vi "FP RT main.vi"() -> ()   [LabVIEW 2014]
uses:
  <vilib>/userdefined/High Color/IMAQdx.ctl
  <vilib>/myRIO/Instrument Drivers/Onboard IO/PWM/typedefs/PWM Reference.ctl
  <vilib>/myRIO/Common/Instrument Driver Framework/Utilities/typedefs/myRIO Generic Hardware Reference.ctl
  <vilib>/myRIO/Common/Instrument Driver Framework/Utilities/typedefs/Hardware Version Enum.ctl
  <vilib>/myRIO/Common/Instrument Driver Framework/Utilities/typedefs/myRIO v1.0 Reference.ctl
  <vilib>/myRIO/Common/Instrument Driver Framework/Utilities/typedefs/Generic FPGA Reference.ctl
  <vilib>/myRIO/Common/Instrument Driver Framework/myRIO v1.0/PWM/typedefs/PWM Channels Enum.ctl
  <vilib>/myRIO/Instrument Drivers/Onboard IO/PWM/typedefs/PWM Configuration.ctl
  <vilib>/userdefined/High Color/nirio_resource_hc.ctl
  <vilib>/myRIO/Instrument Drivers/Onboard IO/DIO/typedefs/DIO Reference.ctl
  <vilib>/myRIO/Common/Instrument Driver Framework/myRIO v1.0/DIO/typedefs/DIO Channels List.ctl
  <vilib>/myRIO/Common/Instrument Driver Framework/myRIO v1.0/DIO/typedefs/DIO Channels Enum.ctl
  <vilib>/myRIO/Instrument Drivers/Onboard IO/AI/typedefs/AI Reference.ctl
  <vilib>/myRIO/Common/Instrument Driver Framework/myRIO v1.0/AI/typedefs/AI Channels List.ctl
  <vilib>/myRIO/Common/Instrument Driver Framework/myRIO v1.0/AI/typedefs/AI Channels Enum.ctl
  <vilib>/myRIO/Common/Instrument Driver Framework/Utilities/typedefs/Analog Scaling Constants List.ctl
  <vilib>/myRIO/Common/Instrument Driver Framework/Utilities/typedefs/Analog Scaling Constants.ctl
  <vilib>/myRIO/Common/Instrument Driver Framework/myRIO v1.0/PWM/vis/myRIO v1.1 Open PWM.vi
  <vilib>/myRIO/Common/Instrument Driver Framework/myRIO v1.0/DIO/vis/myRIO v1.1 Open DIO.vi
  <vilib>/myRIO/Common/Instrument Driver Framework/myRIO v1.0/AI/vis/myRIO v1.1 Open AI.vi
  <vilib>/myRIO/Common/Instrument Driver Framework/Utilities/vis/Validate Channels.vi
  <vilib>/myRIO/Common/Instrument Driver Framework/myRIO v1.0/PWM/vis/myRIO v1.0 Reserve PWM.vi
  <vilib>/myRIO/Common/Instrument Driver Framework/myRIO v1.0/DIO/vis/myRIO v1.0 Reserve DIO.vi
  <vilib>/myRIO/Common/Instrument Driver Framework/myRIO v1.0/AI/vis/myRIO v1.0 Reserve AI.vi
  <vilib>/myRIO/Common/Instrument Driver Framework/myRIO v1.0/PWM/vis/myRIO v1.0 Close PWM.vi
  <vilib>/myRIO/Common/Instrument Driver Framework/myRIO v1.0/DIO/vis/myRIO v1.0 Close DIO.vi
  <vilib>/myRIO/Common/Instrument Driver Framework/myRIO v1.0/AI/vis/myRIO v1.0 Close AI.vi
  <vilib>/myRIO/Common/Instrument Driver Framework/myRIO v1.0/PWM/vis/myRIO v1.0 Build MUX Configuration PWM.vi
  <vilib>/myRIO/Common/Instrument Driver Framework/myRIO v1.0/Resource Manager/vis/myRIO v1.0 Reserve Channel List.vi
  <vilib>/myRIO/Common/Instrument Driver Framework/myRIO v1.0/DIO/vis/myRIO v1.0 Build MUX Configuration DIO.vi
  <vilib>/myRIO/Common/Instrument Driver Framework/myRIO v1.0/AI/vis/myRIO v1.0 Build MUX Configuration AI.vi
  <vilib>/myRIO/Common/Instrument Driver Framework/myRIO v1.0/PWM/vis/myRIO v1.0 Unreserve PWM.vi
  <vilib>/myRIO/Common/Instrument Driver Framework/myRIO v1.0/DIO/vis/myRIO v1.0 Unreserve DIO.vi
  <vilib>/myRIO/Common/Instrument Driver Framework/myRIO v1.0/AI/vis/myRIO v1.0 Unreserve AI.vi
  <vilib>/myRIO/Common/Instrument Driver Framework/myRIO v1.0/Resource Manager/vis/myRIO v1.0 Create Configuration List.vi
  <vilib>/myRIO/Common/Instrument Driver Framework/myRIO v1.0/Resource Manager/vis/myRIO v1.0 Reserve Channel.vi
  <vilib>/myRIO/Common/Instrument Driver Framework/myRIO v1.0/Resource Manager/vis/myRIO v1.0 Unreserve Channel.vi
  <vilib>/myRIO/Common/Instrument Driver Framework/myRIO v1.0/Resource Manager/vis/myRIO v1.0 Unreserve Channel List.vi
  <vilib>/myRIO/Common/Instrument Driver Framework/myRIO v1.0/Resource Manager/vis/myRIO v1.0 Build Mutex Name.vi
  <vilib>/Utility/VariantDataType/GetNumericInfo.vi
  <vilib>/Utility/error.llb/Error Cluster From Error Code.vi
  <vilib>/myRIO/Common/Instrument Driver Framework/myRIO v1.0/myRIO v1.1 Open.vi
  <vilib>/myRIO/Common/Instrument Driver Framework/myRIO v1.0/AI/vis/myRIO v1.0 Get Scaling Constants AI.vi
  <vilib>/myRIO/Common/Instrument Driver Framework/Utilities/vis/IO Manager.vi
  <vilib>/myRIO/Common/Instrument Driver Framework/Utilities/vis/Configuration Manager.vi
  <vilib>/myRIO/Common/Instrument Driver Framework/myRIO v1.0/myRIO v1.0 Close.vi
  <vilib>/myRIO/Common/Instrument Driver Framework/myRIO v1.0/Resource Manager/vis/myRIO v1.0 Configure IO.vi
  <vilib>/myRIO/Common/Instrument Driver Framework/myRIO v1.0/AI/vis/myRIO v1.0 Read AI.vi
  <vilib>/myRIO/Common/Instrument Driver Framework/myRIO v1.0/DIO/vis/myRIO v1.0 Write DIO.vi
  <vilib>/myRIO/Common/Instrument Driver Framework/myRIO v1.0/PWM/vis/myRIO v1.0 Write PWM.vi
  <vilib>/myRIO/Common/Instrument Driver Framework/myRIO v1.0/PWM/vis/myRIO v1.0 Shutdown PWM.vi
  <vilib>/myRIO/Common/Instrument Driver Framework/myRIO v1.0/DIO/vis/myRIO v1.0 Shutdown DIO.vi
  <vilib>/myRIO/Instrument Drivers/Onboard IO/AI/vis/myRIO AI Open.xnode
  <vilib>/myRIO/Instrument Drivers/Onboard IO/DIO/vis/myRIO DIO Open.xnode
  <vilib>/myRIO/Instrument Drivers/Onboard IO/PWM/vis/myRIO PWM Open.xnode
  <vilib>/vision/driver/NI_Vision_Acquisition_Software.lvlib
  <vilib>/myRIO/Instrument Drivers/Onboard IO/AI/AI.lvlib
  <vilib>/myRIO/Instrument Drivers/Onboard IO/DIO/DIO.lvlib
  <vilib>/myRIO/Instrument Drivers/Onboard IO/PWM/PWM.lvlib
panel:
  in  "Tab Control":T1(tab)
  out "BW Image":T2(plugin-control)
  in  "stop":bool
  out "Midbrain?":bool
  out "Rudder":dbl(knob) min=-45.0 max=45.0 step=1.0 scale=-45.0..45.0
  out "Speed":dbl(knob) min=-9.0 max=9.0 step=1.0 scale=-50.0..50.0
  out "Hindbrain?":bool
  out "Forebrain?":bool
  out "Battery Dead?":bool
  out "Complete?":bool=TRUE
  out "Arbiter Graph":cluster{dbl, dbl, dbl[]}(graph)
  in  "Session In":T3="cam0"
  out "Color Image":T2(plugin-control)
  out "Nb Circles":i32
  out "UDP Time Out?":bool
  in  "Tug letter":string="G"
  in  "Run?":bool
  in  "MSpeed":dbl(slide) scale=-50.0..50.0 scale format="%#.1g"
  in  "MHeading":dbl(slide) scale=-45.0..45.0 scale format="%_1f"
  in  "Manual?":bool
  out "Camera Data":T4(array[cluster])
  out "Boat Status":T5={"GPS"={"X pos"=0, "Y pos"=0, "Heading"=0.0}, "IR Sensors"=[{"Name"="Bow", "Angle"=0.0, "Distance"=0.0}], "MOT BAT"=7.2, "RIO BAT"=7.2}
  out "GPS?":bool
  out "Act Com":T6
  out "Forebrain ACT":dbl[](array[numeric])
  out "IR Sensors":T7(array[cluster])
  out "GPS":cluster{"X pos":i32, "Y pos":i32, "Heading":dbl}
  out "RED LED":bool
  out "GREEN LED":bool
  out "BLUE LED":bool
  in  "MDF":T8(array[cluster])=[{"Type"=enum."Start", "X"=250, "Y"=250, "Speed"=0, "Behaviors"=enum."Open Water Transit"}, {"Type"=enum."Waypoint", "X"=400, "Y"=100, "Speed"=20, "Behaviors"=enum."P-Wall Follow"}, {"Type"=enum."Waypoint", "X"=250, "Y"=250, "Speed"=20, "Behaviors"=enum."Open Water Transit"}, {"Type"=enum."Waypoint", "X"=250, "Y"=400, "Speed"=20, "Behaviors"=enum."Open Water Transit"}, {"Type"=enum."Waypoint", "X"=100, "Y"=400, "Speed"=20, "Behaviors"=enum."Open Water Transit"}, {"Type"=enum."End", "X"=250, "Y"=250, "Speed"=0, "Behaviors"=enum."Open Water Transit"}]
  out "Invalid Pos?":bool
  out "error out":errorcluster
  out "Forebrain Comd":T9
  out "size(s)":i32
  out "MDF Active":T8(array[cluster])
  # "To start the Tug, press the \">\" key in the tool bar.\n\nPress the Run? control to start the Mission.\n\nWhen complete the Complete? indicator will light.\n\nIf the Run? is not pressed again, the mission will start again.\n\nAlways press the STOP button to end the operation!!!!!!!!!!!!!"
  # "Press the Manual? button to control\nthe Tug from the sliders"
  # "Stuck indicates that\nthe boat is not moving."
  # "Enter the Letter\nof  your Tug"
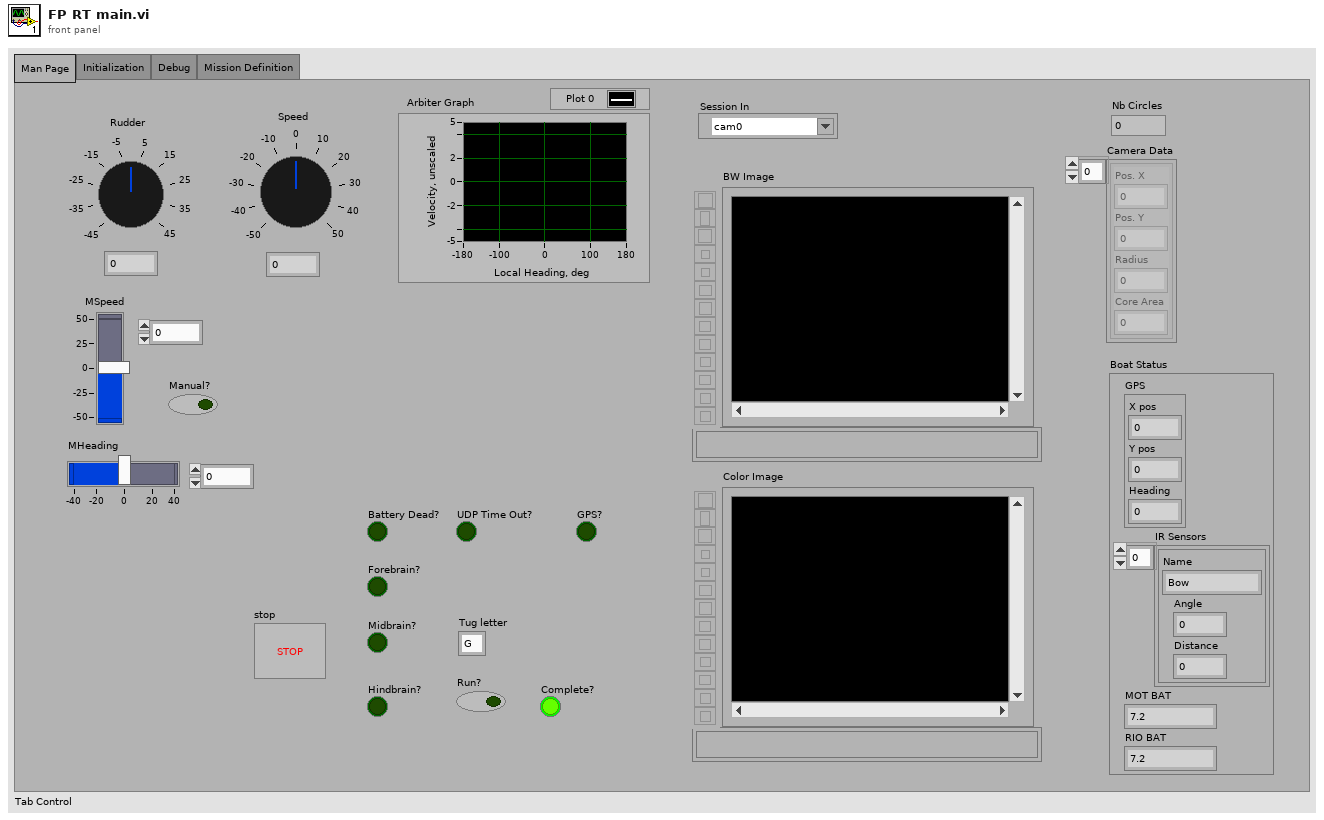
[diagram p1: front panel]
types:
  T1 = enum32{"Man Page", "Initialization", "Debug", "Mission Definition"}
  T2 = typedef "IMAQ Image.ctl" = refnum<image>
  T3 = typedef "IMAQdx.ctl" = refnum<k21>
  T4 = cluster{"Pos. X":i32, "Pos. Y":i32, "Radius":i32, "Core Area":i32}[]
  T5 = cluster{"GPS":cluster{"X pos":i32, "Y pos":i32, "Heading":dbl}, "IR Sensors":cluster{"Name":string, "Angle":dbl, "Distance":dbl}[], "MOT BAT":dbl, "RIO BAT":dbl}
  T6 = cluster{"Desired Local\nHeading":dbl, "Desired\nSpeed":dbl}
  T7 = cluster{"Name":string, "Angle":dbl, "Distance":dbl}[]
  T8 = cluster{"Type":enum16{"Start", "Waypoint", "End"}, "X":i32, "Y":i32, "Speed":i32, "Behaviors":enum16{"Open Water Transit", "P-Wall Follow", "S-Wall Follow", "Dock"}}[]
  T9 = cluster{"Behaviors":enum16{"Open Water Transit", "P-Wall Follow", "S-Wall Follow", "Dock"}, "Behavior\nVelocity":dbl}
  T10 = typedef "nirio_resource_hc.ctl" = tag
  T11 = typedef "Hardware Version Enum.ctl" = enum16{"Unknown", "myRIO-1900", "myRIO-1950"}
  T12 = typedef "Image Type" = u32
  T13 = enum16{"Open Water Transit", "P-Wall Follow", "S-Wall Follow", "Dock"}
  T14 = typedef "PWM.lvlib/PWM Reference.ctl" = cluster{"myRIO Reference":T15, "PWM Channels Enum":T18, "PWM Configuration":T19}
  T15 = typedef "myRIO Generic Hardware Reference.ctl" = cluster{"myRIO Model":T11, "myRIO Hardware Reference":T16}
  T16 = typedef "myRIO v1.0 Reference.ctl" = cluster{"Generic FPGA Reference":T17, "Allow multiple opens":bool}
  T17 = typedef "Generic FPGA Reference.ctl" = refnum<k20>
  T18 = typedef "PWM Channels Enum.ctl" = enum16{"Not Connected", "C/PWM0", "C/PWM1", "A/PWM0", "A/PWM1", "A/PWM2", "B/PWM0", "B/PWM1", "B/PWM2"}
  T19 = typedef "PWM.lvlib/PWM Configuration.ctl" = cluster{"Frequency":dbl, "Duty Cycle":dbl}
  T20 = typedef "DIO.lvlib/DIO Reference.ctl" = cluster{"myRIO Reference":T15, "DIO Channels List":T21}
  T21 = typedef "DIO Channels List.ctl" = T22[]
  T22 = typedef "DIO Channels Enum.ctl" = enum16{"Not Connected", "C/DIO0", "C/DIO1", "C/DIO2", "C/DIO3", "C/DIO4", "C/DIO5", "C/DIO6", "C/DIO7", "A/DIO0", "A/DIO1", "A/DIO2", "A/DIO3", "A/DIO4", "A/DIO5", "A/DIO6", "A/DIO7", "A/DIO8", "A/DIO9", "A/DIO10", "A/DIO11", "A/DIO12", "A/DIO13", "A/DIO14", "A/DIO15", "B/DIO0", "B/DIO1", "B/DIO2", "B/DIO3", "B/DIO4", "B/DIO5", "B/DIO6", "B/DIO7", "B/DIO8", "B/DIO9", "B/DIO10", "B/DIO11", "B/DIO12", "B/DIO13", "B/DIO14", "B/DIO15", "LED0", "LED1", "LED2", "LED3", "Button0"}
  T23 = typedef "AI.lvlib/AI Reference.ctl" = cluster{"myRIO Reference":T15, "AI Channels List":T24, "AI Scaling Constants List":T26}
  T24 = typedef "AI Channels List.ctl" = T25[]
  T25 = typedef "AI Channels Enum.ctl" = enum16{"Not Connected", "AudioIn/Left", "AudioIn/Right", "C/AI0", "C/AI1", "A/AI0", "A/AI1", "A/AI2", "A/AI3", "B/AI0", "B/AI1", "B/AI2", "B/AI3"}
  T26 = typedef "Analog Scaling Constants List.ctl" = T27[]
  T27 = typedef "Analog Scaling Constants.ctl" = cluster{"LSB Weight (Volts)":dbl, "Offset (Volts)":dbl, "Signed?":bool}
  T28 = cluster{"Obs Avoid Array":dbl[], "P-Wall Array":dbl[], "S-Wall Array":dbl[], "Unstuck Array":dbl[]}
  T29 = cluster{"regular expression":string, i32, i32, i32}
  T30 = cluster{"Behaviors":enum16{"Open Water Transit", "P-Wall Follow", "S-Wall Follow", "Dock"}, dbl}
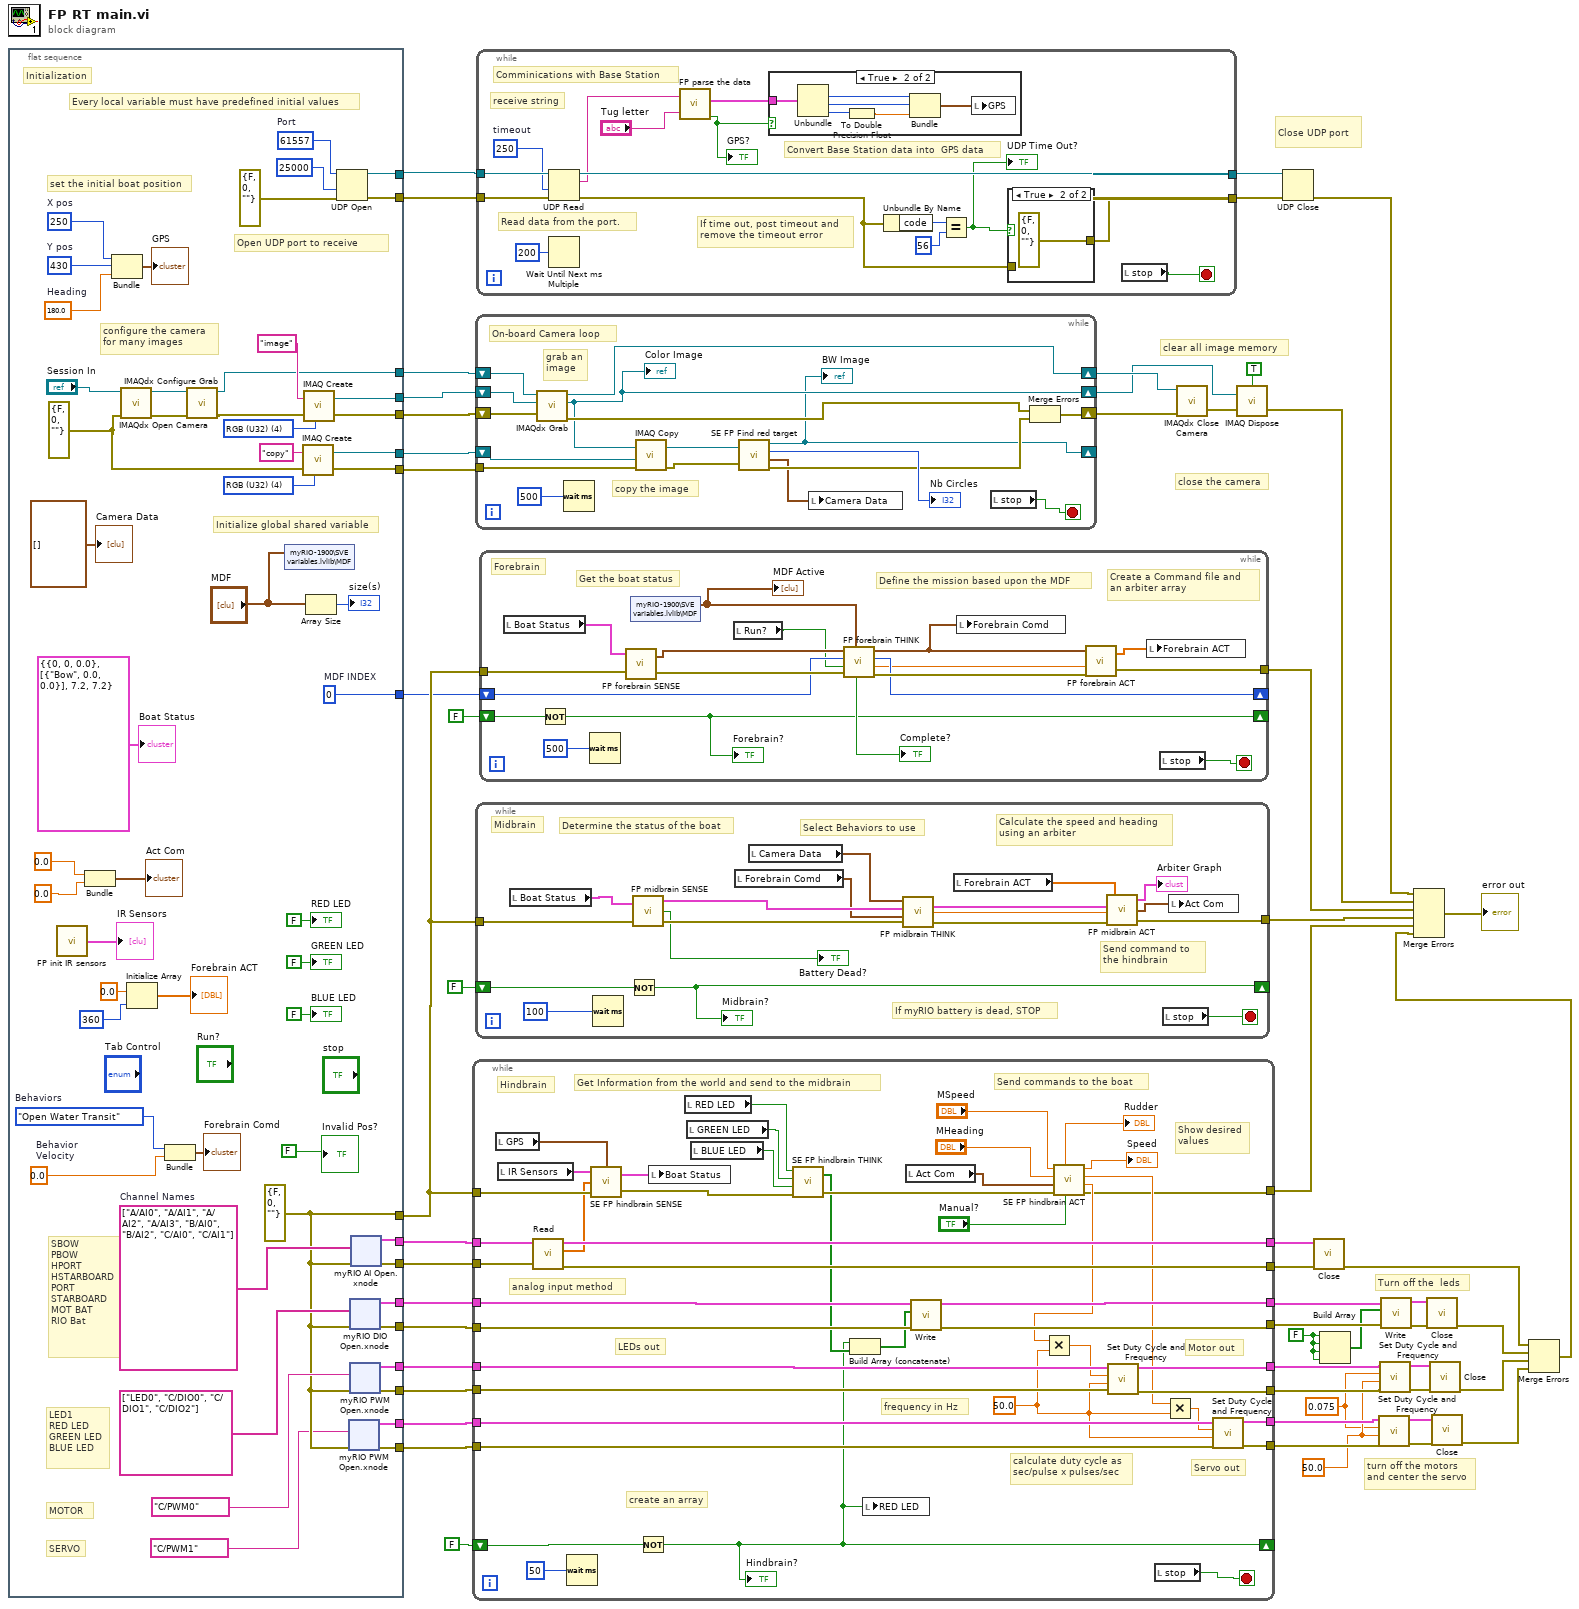
[diagram p0: block diagram]
diagram:
  w2 = 0.075
  w1 = FALSE
  w3 = 50.0
  # "Turn off the  leds"
  # "turn off the motors\nand center the servo"
  # "Close UDP port"
  # "clear all image memory"
  # "close the camera"
  n1 = flat-sequence {
    tunnel: [w68] -> w51
    tunnel: [w103] -> w48
    tunnel: [w94] -> w47
    tunnel: [w93] -> w46
    tunnel: [w92] -> w45
    tunnel: [w88] -> w38
    tunnel: [w87] -> w39
    tunnel: [w83] -> w33
    tunnel: [w82] -> w34
    tunnel: [w76] -> w31
    tunnel: [w75] -> w30
    tunnel: [w73] -> w26
    tunnel: [w72] -> w27
    tunnel: [w70] -> w25
    tunnel: [w69] -> w24
    tunnel: [w66] -> w23
    tunnel: [w65] -> w22
    frame #0 {
      w77 = tag[] ["A/AI0", "A/AI1", "A/AI2", "A/AI3", "B/AI0", "B/AI2", "C/AI0", "C/AI1"]  # Channel Names
      w79 = 430  # Y pos
      w80 = 250  # X pos
      w81 = 180.0  # Heading
      w86 = u16 61557  # Port
      w91 = T12 4 items=["Grayscale (U8)", "Grayscale (I16)", "Grayscale (SGL)", "Complex (CSG)", "RGB (U32)", "HSL (U32)", "RGB (U64)", "Grayscale (U16)"] ("Image Type")
      w89 = errorcluster {"status"=FALSE, "code"=0, "source"=""} ("error in")
      w99 = T12 4 items=["Grayscale (U8)", "Grayscale (I16)", "Grayscale (SGL)", "Complex (CSG)", "RGB (U32)", "HSL (U32)", "RGB (U64)", "Grayscale (U16)"] ("Image Type")
      w68 = errorcluster {"status"=FALSE, "code"=0, "source"=""} ("error out")
      w103 = 0  # MDF INDEX
      w107 = 0.0  # Behavior Velocity
      w102 = T13."Open Water Transit"  # Behaviors
      # "Initialize global shared variable"
      # "LED1\nRED LED\nGREEN LED\nBLUE LED"
      # "SERVO"
      # "MOTOR"
      # "SBOW\nPBOW\nHPORT\nHSTARBOARD\nPORT\nSTARBOARD\nMOT BAT\nRIO Bat"
      # "set the initial boat position"
      # "Open UDP port to receive"
      # "configure the camera\nfor many images"
      # "Every local variable must have predefined initial values"
      # "Initialization"
      n2 = call "FP init IR sensors.vi"() -> ("IR Sensors"=→"IR Sensors":T7)  [unwired: 1 in]
      n3 = Bundle(0.0, 0.0) -> (→"Act Com":cluster{dbl, dbl})  [unwired: 1 in]
      n4 = Bundle("X pos"=w80, "Y pos"=w79, "Heading"=w81) -> (→"GPS":cluster{"X pos":i32, "Y pos":i32, "Heading":dbl})  [unwired: 1 in]
      n5 = call <vilib>:"IMAQdx Open Camera.vi"("error in"=w89, "Session In"="Session In") -> ("error out"=w96:errorcluster, "Session Out"=w95:T3)  [unwired: 1 in, 7 out]
      n6 = Initialize Array(0.0 ("element"), 360 ("dimension size")) -> (→"Forebrain ACT":dbl[])
      n7 = Bundle("Behaviors"=w102, "Behavior\nVelocity"=w107) -> (→"Forebrain Comd":T9)  [unwired: 1 in]
      n8 = call <vilib>:"IMAQdx Configure Grab.vi"("error in"=w96, "Session In"=w95) -> ("error out"=w100:errorcluster, "Session Out"=w92:T3)  [unwired: 8 out]
      n9 = shared-variable "myRIO-1900\\SVE variables.lvlib\\MDF"("MDF") -> ()  [unwired: 1 in, 1 out]
      n10 = call "IMAQ Create"("Image Name"="copy", "Image Type"=w91, "error in (no error)"=w89) -> ("New Image"=w87:T2, "error out"=w88:errorcluster)  [unwired: 2 in]
      n11 = call "IMAQ Create"("Image Name"="image", "Image Type"=w99, "error in (no error)"=w100) -> ("New Image"=w93:T2, "error out"=w94:errorcluster)  [unwired: 1 in, 1 out]
      n12 = Array Size(array="MDF") -> (size(s)=→"size(s)":i32)
      n13 = UDP Open(8:errorcluster {"status"=FALSE, "code"=0, "source"=""} ("error in"), 9:25000 ("timeout ms (25000)"), 11:w86) -> (port=w83:refnum<k16>, 0:w82:errorcluster)  [unwired: 2 in, 1 out]
      n14 = xnode "myRIO PWM Open.xnode"("error in (no error)"=w68, "Channel Name"=tag "C/PWM1") -> ("error out"=w66:errorcluster, "PWM Ref Out"=w65:T14)  [unwired: 1 in]
      n15 = xnode "myRIO DIO Open.xnode"("error in (no error)"=w68, "Channel Names"=tag[] ["LED0", "C/DIO0", "C/DIO1", "C/DIO2"]) -> ("error out"=w73:errorcluster, "DIO Ref Out"=w72:T20)  [unwired: 1 in]
      n16 = xnode "myRIO PWM Open.xnode"("error in (no error)"=w68, "Channel Name"=tag "C/PWM0") -> ("error out"=w70:errorcluster, "PWM Ref Out"=w69:T14)  [unwired: 1 in]
      n17 = xnode "myRIO AI Open.xnode"("error in (no error)"=w68, "Channel Names"=w77) -> ("error out"=w76:errorcluster, "AI Ref Out"=w75:T23)  [unwired: 1 in]
      "Invalid Pos?" <- FALSE
      "RED LED" <- FALSE ("RED LED")
      "GREEN LED" <- FALSE ("GREEN LED")
      "BLUE LED" <- FALSE ("WHITE LED")
      "Camera Data" <- T4 [] ("Camera Data")
      "Boat Status" <- T5 {"GPS"={"X pos"=0, "Y pos"=0, "Heading"=0.0}, "IR Sensors"=[{"Name"="Bow", "Angle"=0.0, "Distance"=0.0}], "MOT BAT"=7.2, "RIO BAT"=7.2} ("Boat Status 2")
    }
  }
  n18 = while {
    tunnel: w51 -> [w218]
    tunnel: [w191] -> w55
    shift-right: [w179] -> _
    shift-left: FALSE -> [w206]
    tunnel: w31 -> [w214]
    tunnel: w30 -> [w213]
    tunnel: [w212] -> w29
    tunnel: [w211] -> w28
    tunnel: w27 -> [w209]
    tunnel: w26 -> [w210]
    tunnel: [w208] -> w8
    tunnel: [w207] -> w5
    tunnel: w25 -> [w204]
    tunnel: w24 -> [w205]
    tunnel: [w203] -> w17
    tunnel: [w202] -> w14
    tunnel: w23 -> [w201]
    tunnel: [w200] -> w21
    tunnel: w22 -> [w199]
    tunnel: [w198] -> w19
    stop <- w220 stop-if-true
    w193 = 50.0
    # "create an array"
    # "frequency in Hz"
    # "calculate duty cycle as\nsec/pulse x pulses/sec"
    # "Show desired\nvalues"
    # "Motor out"
    # "Servo out"
    # "LEDs out"
    # "analog input method"
    # "Send commands to the boat"
    # "Get Information from the world and send to the midbrain"
    # "Hindbrain"
    n19 = local read "GPS"() -> (w215:cluster{"X pos":i32, "Y pos":i32, "Heading":dbl})
    n20 = local read "IR Sensors"() -> (w217:T7)
    n21 = call <vilib>:"Read.vi"("error in (no error)"=w214, "AI Ref In"=w213) -> ("error out"=w212:errorcluster, "Values"=w197:dbl[], "AI Ref Out"=w211:T23)  [unwired: 7 in]
    n22 = Wait (ms)(milliseconds to wait=u32 50) -> ()  [unwired: 1 out]
    n23 = call "SE FP hindbrain SENSE.vi"("GPS"=w215, "error in"=w218, "Analog Input Values"=w197, "IR Sensors"=w217) -> ("error out"=w216:errorcluster, "Boat Status"=w178:T5)
    n24 = Not(x=w206) -> (.not. x?=w179:bool)
    "Hindbrain?" <- w179
    n25 = local write "Boat Status"(w178) -> ()
    n26 = local read "RED LED"() -> (w182:bool)
    n27 = local read "GREEN LED"() -> (w181:bool)
    n28 = local read "BLUE LED"() -> (w180:bool)
    n29 = call "SE FP hindbrain THINK.vi"("error in"=w216, "BLUE LED"=w180, "GREEN LED"=w181, "RED LED"=w182) -> ("error out"=w191:errorcluster, "LED array"=w184:bool[])
    n30 = Build Array (concatenate)(w179, w184) -> (w183:bool[])
    n31 = local write "RED LED"(w179) -> ()
    n32 = local read "Act Com"() -> (w188:T6)
    n33 = call <vilib>:"Write.vi"("error in (no error)"=w210, "Values"=w183, "DIO Ref In"=w209) -> ("error out"=w208:errorcluster, "DIO Ref Out"=w207:T20)  [unwired: 6 in]
    n34 = call "SE FP hindbrain ACT.vi"("Manual?"="Manual?", "error in"=w191, "Act Com"=w188, "MHeading"="MHeading", "MSpeed"="MSpeed") -> ("Speed"=w196:dbl, "Rudder"=w194:dbl, "Desired\nSpeed"=→"Speed":dbl, "Desired \nRudder"=→"Rudder":dbl)  [unwired: 1 out]
    n35 = Multiply(x=w196, y=w193) -> (x*y=w195:dbl)
    n36 = call <vilib>:"Set Duty Cycle and Frequency.vi"("error in (no error)"=w204, "Frequency [Hz]"=w193, "Duty Cycle"=w195, "PWM Ref In"=w205) -> ("error out"=w203:errorcluster, "PWM Ref Out"=w202:T14)  [unwired: 5 in]
    n37 = local read "stop"() -> (w220:bool)
    n38 = Multiply(x=w194, y=w193) -> (x*y=w192:dbl)
    n39 = call <vilib>:"Set Duty Cycle and Frequency.vi"("error in (no error)"=w201, "Frequency [Hz]"=w193, "Duty Cycle"=w192, "PWM Ref In"=w199) -> ("error out"=w200:errorcluster, "PWM Ref Out"=w198:T14)  [unwired: 5 in]
  }
  n40 = while {
    shift-right: [w224] -> w43
    shift-left: w47 -> [w236]
    shift-right: [w223] -> w41
    shift-left: w46 -> [w235]
    shift-right: [w228] -> w42
    shift-left: w45 -> [w234]
    tunnel: w38 -> [w232]
    shift-right: [w222] -> _
    shift-left: w39 -> [w231]
    stop <- w237 stop-if-true
    # "grab an\nimage"
    # "copy the image"
    # "On-board Camera loop"
    n41 = call <vilib>:"IMAQdx Grab.vi"("error in"=w236, "Image In"=w235, "Session In"=w234) -> ("error out"=w225:errorcluster, "Image Out"=w223:T2, "Session Out"=w228:T3)  [unwired: 5 in, 1 out]
    "Color Image" <- w223
    n42 = Wait (ms)(milliseconds to wait=u32 500) -> ()  [unwired: 1 out]
    n43 = call "IMAQ Copy"("error in (no error)"=w232, "Image Dst"=w231, "Image Src"=w223) -> ("error out"=w230:errorcluster, "Image Dst Out"=w229:T2)  [unwired: 3 in]
    n44 = call "SE FP Find red target.vi"("Image In"=w229, "error in (no error)"=w230) -> ("Image Dst Out"=w222:T2, "Nb Circles (Circle Detection 1)"=→"Nb Circles":i32, "Camera Data"=w221:T4, "error out"=w226:errorcluster)
    "BW Image" <- w222
    n45 = local write "Camera Data"(w221) -> ()
    n46 = local read "stop"() -> (w237:bool)
    n47 = Merge Errors(w225, w226) -> (w224:errorcluster)
  }
  n48 = while {
    shift-right: [w243] -> _
    shift-left: FALSE -> [w254]
    tunnel: w51 -> [w253]
    tunnel: [w247] -> w53
    stop <- w255 stop-if-true
    # "If myRIO battery is dead, STOP"
    # "Send command to \nthe hindbrain"
    # "Calculate the speed and heading\nusing an arbiter"
    # "Select Behaviors to use"
    # "Determine the status of the boat"
    # "Midbrain"
    n49 = local read "Boat Status"() -> (w238:T5)
    n50 = Wait (ms)(milliseconds to wait=u32 100) -> ()  [unwired: 1 out]
    n51 = Not(x=w254) -> (.not. x?=w243:bool)
    "Midbrain?" <- w243
    n52 = call "FP midbrain SENSE.vi"("Boat Status"=w238, "error in"=w253) -> ("IR Sensors"=w241:T7, "Battery\nDead?"=→"Battery Dead?":bool, "error out"=w251:errorcluster)
    n53 = local read "Forebrain Comd"() -> (w240:T9)
    n54 = local read "Camera Data"() -> (w239:T4)
    n55 = call "FP midbrain THINK.vi"("error in"=w251, "Forebrain Comd"=w240, "IR Sensors"=w241, "Camera Data"=w239) -> ("error out"=w250:errorcluster, "Behavior\nVelocity OUT"=w245:dbl, "Behavior arrays"=w248:T28)
    n56 = local read "Forebrain ACT"() -> (w246:dbl[])
    n57 = call "FP midbrain ACT.vi"("error in"=w250, "Behavior\nVelocity"=w245, "Behavior arrays"=w248, "Forebrain ACT"=w246) -> ("error out"=w247:errorcluster, "Act Com"=w252:T6, "Waveform Graph"=→"Arbiter Graph":cluster{dbl, dbl, dbl[]})
    n58 = local read "stop"() -> (w255:bool)
    n59 = local write "Act Com"(w252) -> ()
  }
  n60 = while {
    tunnel: w34 -> [w270]
    tunnel: w33 -> [w269]
    tunnel: [w268] -> w36
    tunnel: [w263] -> w35
    stop <- w260 stop-if-true
    w262 = 250  # timeout
    # "Convert Base Station data into  GPS data"
    # "Comminications with Base Station"
    # "receive string"
    # "If time out, post timeout and\nremove the timeout error"
    # "Read data from the port."
    n61 = UDP Read(connection ID=w269, timeout ms (25000)=w262, 8:w270) -> (data out=w257:string, error out=w264:errorcluster, 3:w268:refnum<k16>)  [unwired: 1 in, 2 out]
    n62 = Wait Until Next ms Multiple(millisecond multiple=u32 200) -> ()  [unwired: 1 out]
    n63 = call "FP parse the data.vi"("Nav String"=w257, "Tug"="Tug letter") -> ("Tug Location"=w258:T29, "Valid?"=w256:bool)  [unwired: 2 out]
    "GPS?" <- w256
    n64 = case shown="True" w256 {
      tunnel: w258 -> [_ w276]
      frame False {
      }
      frame True {
        n65 = Unbundle(w276) -> (w275:i32, w274:i32, w272:i32)  [unwired: 1 out]
        n66 = To Double Precision Float(number=w272) -> (double precision float=w273:dbl)
        n67 = Bundle(w275, w274, w273) -> (w271:cluster{i32, i32, dbl})  [unwired: 1 in]
        n68 = local write "GPS"(w271) -> ()
      }
    }
    n69 = Unbundle By Name(w264) -> ("code"=w267:i32)
    n70 = Equal?(x=w267, y=56) -> (x = y?=w265:bool)
    "UDP Time Out?" <- w265
    n71 = case shown="True" w265 {
      tunnel: [w277 errorcluster {"status"=FALSE, "code"=0, "source"=""} ("error out")] -> w263
      tunnel: w264 -> [w277 _]
      frame False {
      }
      frame True {
      }
    }
    n72 = local read "stop"() -> (w260:bool)
  }
  n73 = while {
    tunnel: w51 -> [w294]
    shift-right: [w282] -> _
    shift-left: FALSE -> [w283]
    tunnel: [w291] -> w49
    shift-right: [w287] -> _
    shift-left: w48 -> [w285]
    stop <- w295 stop-if-true
    # "Create a Command file and \nan arbiter array"
    # "Define the mission based upon the MDF"
    # "Get the boat status"
    # "Forebrain"
    n74 = local read "Boat Status"() -> (w289:T5)
    n75 = Not(x=w283) -> (.not. x?=w282:bool)
    "Forebrain?" <- w282
    n76 = Wait (ms)(milliseconds to wait=u32 500) -> ()  [unwired: 1 out]
    n77 = call "FP forebrain SENSE.vi"("error in"=w294, "Boat Status"=w289) -> ("error out"=w293:errorcluster, "GPS"=w288:cluster{"X pos":i32, "Y pos":i32, "Heading":dbl})  [unwired: 1 in]
    n78 = shared-variable "myRIO-1900\\SVE variables.lvlib\\MDF"() -> (w279:T8)  [unwired: 1 in, 1 out]
    "MDF Active" <- w279
    n79 = local read "Run?"() -> (w281:bool)
    n80 = call "FP forebrain THINK.vi"("MDF in"=w279, "error in"=w293, "Run?"=w281, "MDF index"=w285, "GPS"=w288) -> ("error out"=w292:errorcluster, "local Steering\nangle"=w286:dbl, "MDF Index out"=w287:i32, "Behaviors out"=w280:T30, "Complete?"=→"Complete?":bool)
    n81 = local write "Forebrain Comd"(w280) -> ()
    n82 = call "FP forebrain ACT.vi"("error in"=w292, "local Steering\nangle"=w286, "Behaviors in"=w280) -> ("error out"=w291:errorcluster, "Forebrain ACT"=w290:dbl[])
    n83 = local write "Forebrain ACT"(w290) -> ()
    n84 = local read "stop"() -> (w295:bool)
  }
  n85 = call <vilib>:"IMAQdx Close Camera.vi"("error in"=w43, "Session In"=w42) -> ("error out"=w44:errorcluster)  [unwired: 9 out]
  n86 = call "IMAQ Dispose"("All Images? (No)"=TRUE, "Image"=w41, "error in (no error)"=w44) -> ("error out"=w40:errorcluster)  [unwired: 3 out]
  n87 = UDP Close(connection ID=w36, 8:w35) -> (error out=w32:errorcluster)  [unwired: 1 out]
  n88 = call <vilib>:"Close.vi"("error in (no error)"=w29, "AI Ref In"=w28) -> ("error out"=w10:errorcluster)  [unwired: 9 in]
  n89 = Build Array(w1, w1, w1, w1) -> (w4:bool[])
  n90 = call <vilib>:"Set Duty Cycle and Frequency.vi"("error in (no error)"=w21, "Frequency [Hz]"=w3, "Duty Cycle"=w2, "PWM Ref In"=w19) -> ("error out"=w20:errorcluster, "PWM Ref Out"=w18:T14)  [unwired: 5 in]
  n91 = call <vilib>:"Set Duty Cycle and Frequency.vi"("error in (no error)"=w17, "Frequency [Hz]"=w3, "Duty Cycle"=w2, "PWM Ref In"=w14) -> ("error out"=w16:errorcluster, "PWM Ref Out"=w15:T14)  [unwired: 5 in]
  n92 = call <vilib>:"Write.vi"("error in (no error)"=w8, "Values"=w4, "DIO Ref In"=w5) -> ("error out"=w7:errorcluster, "DIO Ref Out"=w6:T20)  [unwired: 6 in]
  n93 = call <vilib>:"Close.vi"("error in (no error)"=w7, "DIO Ref In"=w6) -> ("error out"=w11:errorcluster)  [unwired: 9 in]
  n94 = call <vilib>:"Close.vi"("error in (no error)"=w16, "PWM Ref In"=w15) -> ("error out"=w12:errorcluster)  [unwired: 9 in]
  n95 = call <vilib>:"Close.vi"("error in (no error)"=w20, "PWM Ref In"=w18) -> ("error out"=w13:errorcluster)  [unwired: 9 in]
  n96 = Merge Errors(w10, w11, w12, w13) -> (w9:errorcluster)
  n97 = Merge Errors(w32, w40, w49, w53, w55, w9) -> (→"error out":errorcluster)
